vi "Get Optimiser Cell.vi"(8 "error in (no error)":errorcluster, 11 "Run Block in":refnum<class "Run Block.lvclass">) -> (0 "error out":errorcluster, 2 "Optimiser Cell":refnum<class "Optimiser Cell.lvclass">, 3 "Run Block out":refnum<class "Run Block.lvclass">)   [LabVIEW 2020, in "Run Utilities.lvlib" / "Run Block.lvclass"]
doc: "VI for obtaining the first cell in the schedule and casting it into optimiser cell. If the cell is not an optimser cell, this VI will throw errors"
uses:
  Run Block.lvclass
  Optimiser Cell/Optimiser Cell.lvclass
  Ancestor/Ancestor/Ancestor.lvclass/Ancestor.ctl
  Support VIs/Generate Error.vi
  FGV/Error Memory/Get Error Description.vi
  Support VIs/Get PC name.vi
  Ancestor/Ancestor/Read ID.vi
  Support VIs/Get Class Name.vi
  <vilib>/Utility/error.llb/Clear Errors.vi
  FGV/Error Memory/Error Memory Core.vi
  <vilib>/AdvancedString/Delimited String to 1D String Array.vi
  Support VIs/Circus Root Path.vi
  FGV/Error Memory/Error Crt Lvl checker.vi
  FGV/Error Memory/Error Memory Core.vi/40c8088d-b597-4017-91af-faa98e00292e.vi
  FGV/Error Memory/Error Memory Core.vi/d4a3ab98-063c-4e44-b43d-fbdcfe6c2be2.vi
  Support VIs/Global Memory.vi
  <vilib>/Utility/LVClass/Get LV Class Name.vi
  Support VIs/Is in Packed Library.vi
  Support VIs/TALOS Root path.vi
  Support VIs/Read CSV worksheet.vi
  Support VIs/Global Constants.vi
  <vilib>/Utility/error.llb/General Error Handler.vi
  Support VIs/Error Log.vi
  Schedule/Schedule.lvclass
  Ancestor/Ancestor/Ancestor.lvclass
  <vilib>/Comparison/Equal/Equal Functor/Equal Functor.lvclass
  Run Block.lvclass/Run Block.ctl
  TALOS.lvlib
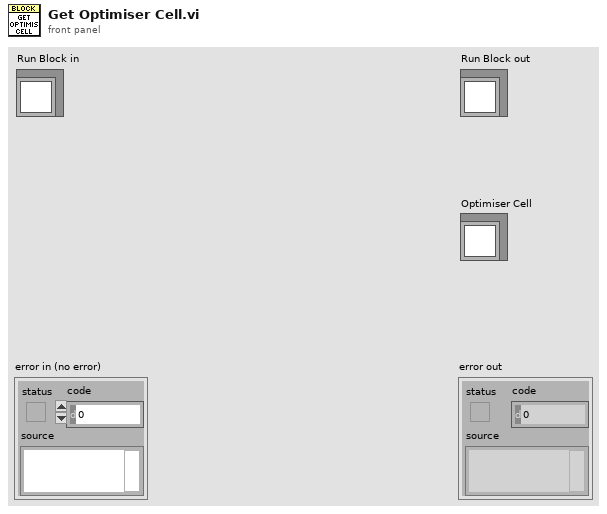
[diagram p1: front panel]
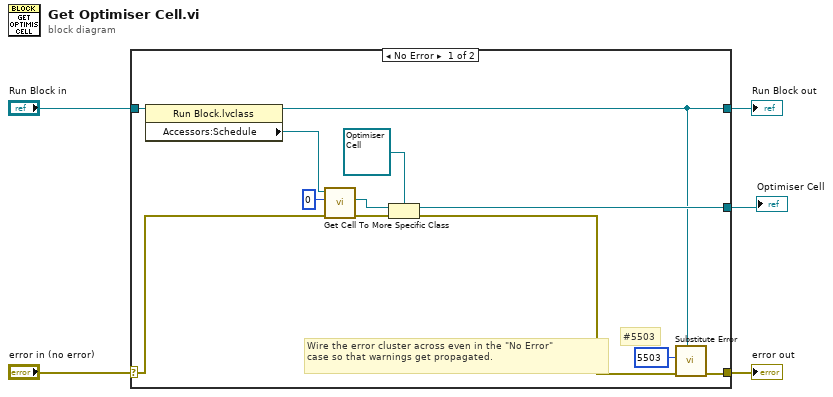
[diagram p0: block diagram]
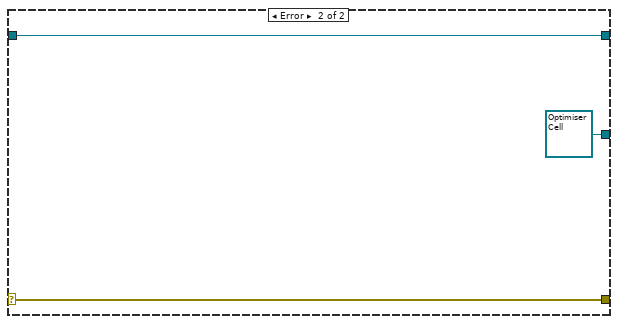
[diagram p2: hidden frame]
diagram:
  n1 = case shown="No Error" "error in (no error)" {
    selector: "error in (no error)" -> [w14 w20]
    tunnel: [w8 w20] -> w4
    tunnel: [w7 w19] -> w2
    tunnel: "Run Block in" -> [w17 w19]
    tunnel: [w10 refnum<class "Optimiser Cell.lvclass"> refnum ("Scheduling.lvlib:Optimiser Cell.lvclass")] -> w1
    frame No Error {
      # "#5503"
      # "Wire the error cluster across even in the \"No Error\"\ncase so that warnings get propagated."
      n2 = property class="Run Block.lvclass"(reference=w17) -> (reference out=w7:refnum<class "Run Block.lvclass">, "Accessors:Schedule"=w16:refnum<class "Schedule.lvclass">)  [unwired: 1 in, 1 out]
      n3 = call-dynamic "Get Cell.vi"("error in (no error)"=w14, "index"=0, "Schedule in"=w16) -> ("error out"=w12:errorcluster, "Schedule Cell"=w13:refnum<class "Schedule Cell.lvclass">)  [unwired: 6 in, 1 out]
      n4 = To More Specific Class(target class=refnum<class "Optimiser Cell.lvclass"> refnum ("Scheduling.lvlib:Optimiser Cell.lvclass"), reference=w13, error in=w12) -> (specific class reference=w10:refnum<class "Optimiser Cell.lvclass">, error out=w9:errorcluster)
      n5 = call "Substitute Error.vi"("LabVIEW Object"=w7, "error in (no error)"=w9, "Error Code"=5503) -> ("error out"=w8:errorcluster)  [unwired: 8 in]
    }
    frame Error {
    }
  }
  "error out" <- w4
  "Run Block out" <- w2
  "Optimiser Cell" <- w1
